vi "Resolve Promise.vi"(8 "error in (no error)":errorcluster, 10 "Value":variant, 11 "Future in":refnum<class "Promise.lvclass">) -> (0 "error out":errorcluster, 3 "Future out":refnum<class "Promise.lvclass">)   [LabVIEW 2017, in "Promise.lvlib" / "Promise.lvclass"]
uses:
  Promise.lvclass
  Promise.lvclass/Promise.ctl
  <vilib>/Utility/error.llb/Error Cluster From Error Code.vi
  <vilib>/ErrorRing/Error Ring.xnode
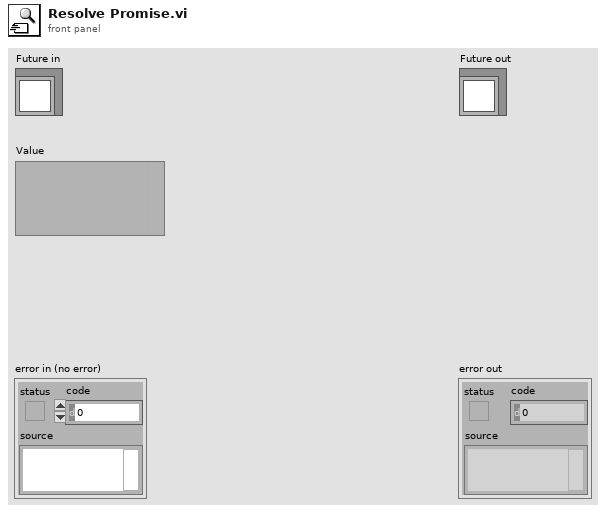
[diagram p1: front panel]
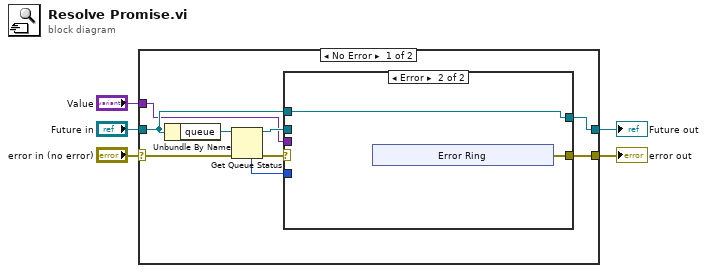
[diagram p0: block diagram]
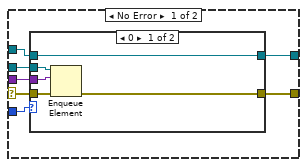
[diagram p2: hidden frame]
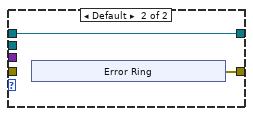
[diagram p3: hidden frame]
diagram:
  n1 = case shown="No Error" "error in (no error)" {
    selector: "error in (no error)" -> [w8 w42]
    tunnel: [w14 w42] -> w4
    tunnel: [w12 w41] -> w2
    tunnel: "Future in" -> [w13 w41]
    tunnel: "Value" -> [w6 _]
    frame No Error {
      n2 = Unbundle By Name(w13) -> ("queue"=w11:refnum<queue>)
      n3 = Get Queue Status(queue=w11, error in (no error)=w8) -> (queue out=w9:refnum<queue>, error out=w7:errorcluster, # elements in queue=w10:i32)  [unwired: 1 in, 5 out]
      n4 = case shown="Error" w7 {
        selector: w7 -> [w16 _]
        tunnel: [w21 w34] -> w14
        tunnel: w13 -> [w20 w35]
        tunnel: [w19 w35] -> w12
        tunnel: w10 -> [w18 _]
        tunnel: w9 -> [w17 _]
        tunnel: w6 -> [w15 _]
        frame No Error {
          n5 = case shown="0" w18 {
            tunnel: w20 -> [w26 w28]
            tunnel: w16 -> [w24 _]
            tunnel: [w23 w27] -> w21
            tunnel: [w26 w28] -> w19
            tunnel: w15 -> [w22 _]
            tunnel: w17 -> [w25 _]
            frame 0 {
              n6 = Enqueue Element(queue=w25, element=w22, error in (no error)=w24) -> (error out=w23:errorcluster)  [unwired: 1 in, 2 out]
            }
            frame Default {
              n7 = xnode "Error Ring"() -> ("error out"=w27:errorcluster)
            }
          }
        }
        frame Error {
          n8 = xnode "Error Ring"() -> ("error out"=w34:errorcluster)
        }
      }
    }
    frame Error {
    }
  }
  "error out" <- w4
  "Future out" <- w2
